vi "Send Message Module.vi"(7 "priority (normal)":T1, 8 "Error In":errorcluster, 9 "Data":variant, 10 "Message":string, 11 "Target ModuleName In":T2=enum."Controller") -> (0 "error in (no error)":errorcluster)   [LabVIEW 2019, in "Architecture.lvlib"]
doc: "This method is used to send an asynchronous message to a target module. It generates a user event that will be handled by target module's event structure."
uses:
  Architecture.lvlib
  Typedefs/Enum_Module_Name.ctl
  <vilib>/event_ctls.llb/usereventprio.ctl
  Typedefs/Module References.ctl
  Typedefs/Message.ctl
  Typedefs/FGV Ref. Modules Function.ctl
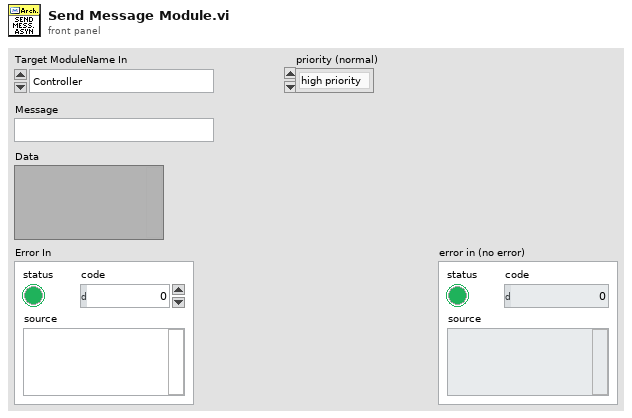
[diagram p1: front panel]
types:
  T1 = typedef "usereventprio.ctl" = enum32{"high priority", "normal priority"}
  T2 = typedef "Architecture.lvlib/Enum_Module_Name.ctl" = enum16{"Configuration", "Error_Handler", "Log", "Database", "Controller", "User Console", "Display Console", "Sensor Interface"}
  T3 = typedef "Architecture.lvlib/Message.ctl" = cluster{"Message":string, "Data":variant, "syn":bool}
  T4 = typedef "Architecture.lvlib/FGV Ref. Modules Function.ctl" = enum16{"Init ", "Add Module", "Get Module", "Get All", "Add Asynchronous Run Ref", "Dispose"}
  T5 = typedef "Architecture.lvlib/Module References.ctl" = cluster{"ModuleName":T2, "Queue":refnum<queue>, "user event":refnum<user-event>, "VI Refnum":refnum<vi>, "ShowFP":bool, "StatesTracking Enabled":bool}
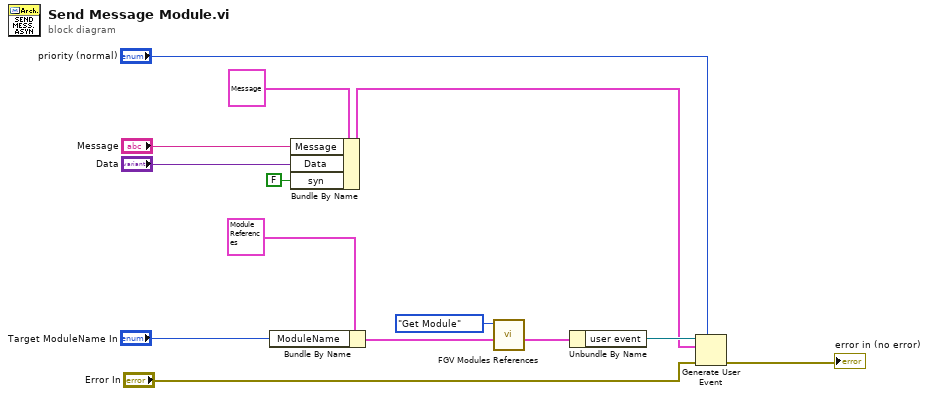
[diagram p0: block diagram]
diagram:
  n1 = Bundle By Name(cluster=T5 {"ModuleName"=enum."Controller", "Queue"=refnum, "user event"=refnum, "VI Refnum"=refnum, "ShowFP"=FALSE, "StatesTracking Enabled"=FALSE} ("Module_Refs"), "ModuleName"="Target ModuleName In") -> (w12:T5)
  n2 = Bundle By Name(cluster=T3 {"Message"="", "Data"=variant, "syn"=FALSE} ("event data"), "Message"="Message", "Data"="Data", "syn"=FALSE) -> (w7:T3)
  n3 = call "FGV Modules References.vi"("Module_Refs"=w12, "FGV Ref. Function In"=FGV_Ref._Modules_Function."Get Module") -> ("Module_Ref Out"=w10:T5)  [unwired: 7 in, 2 out]
  n4 = Unbundle By Name(w10) -> ("user event"=w9:refnum<user-event>)
  n5 = Generate User Event(priority (normal)="priority (normal)", user event=w9, event data cluster=w7, error in="Error In") -> (error out=→"error in (no error)":errorcluster)  [unwired: 1 out]
